vi "處理次數.vi"() -> ()   [LabVIEW 2015]
uses:
  <vilib>/vision/NI_Vision_Development_Module.lvlib
panel:
  out "Count":i32
  in  "Gap":i32=10 min=1 max=300
  in  "Direction":T1(ring)
  in  "Rectangle Points":T2[](array[typedef]) {"Y" format="%.2f"; "X" format="%.2f"}
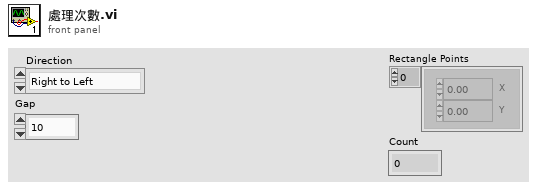
[diagram p1: front panel]
types:
  T1 = enum16{"Right to Left", "Left  to Right", "Up to Down", "Down to Up"}
  T2 = typedef "IMAQ Point" = cluster{"X":sgl, "Y":sgl}
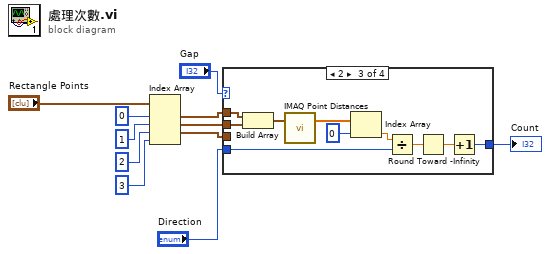
[diagram p0: block diagram]
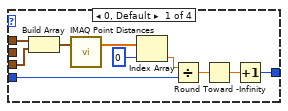
[diagram p2: hidden frame]
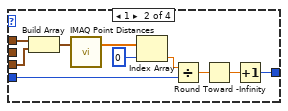
[diagram p3: hidden frame]
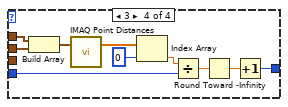
[diagram p4: hidden frame]
diagram:
  n1 = Index Array(array="Rectangle Points", index #1=0 ("index"), index #2=1 ("index"), index #3=2 ("index"), index #4=3 ("index")) -> (element #1=w6:T2, element #2=w4:T2, element #3=w5:T2)  [unwired: 1 out]
  n2 = case shown="2" "Gap" {
    tunnel: "Direction" -> [w19 w29 w39 w49]
    tunnel: [w18 w28 w38 w48] -> w1
    tunnel: w6 -> [w15 w25 w37 w45]
    tunnel: w5 -> [w14 w24 _ _]
    tunnel: w4 -> [_ _ w33 w44]
    frame 0, Default {
      n3 = Build Array(w15, w14) -> (w17:T2[])
      n4 = call "IMAQ Point Distances"("Points"=w17) -> ("Distances"=w16:sgl[])  [unwired: 4 in, 1 out]
      n5 = Index Array(array=w16, index=0) -> (element=w12:sgl)
      n6 = Divide(x=w12, y=w19) -> (x/y=w20:sgl)
      n7 = Round Toward -Infinity(1:w20) -> (0:w21:sgl)
      n8 = Increment(x=w21) -> (x+1=w18:i32)
    }
    frame 1 {
      n9 = Build Array(w25, w24) -> (w27:T2[])
      n10 = call "IMAQ Point Distances"("Points"=w27) -> ("Distances"=w26:sgl[])  [unwired: 4 in, 1 out]
      n11 = Index Array(array=w26, index=0) -> (element=w22:sgl)
      n12 = Divide(x=w22, y=w29) -> (x/y=w30:sgl)
      n13 = Round Toward -Infinity(1:w30) -> (0:w31:sgl)
      n14 = Increment(x=w31) -> (x+1=w28:i32)
    }
    frame 2 {
      n15 = Build Array(w37, w33) -> (w36:T2[])
      n16 = call "IMAQ Point Distances"("Points"=w36) -> ("Distances"=w35:sgl[])  [unwired: 4 in, 1 out]
      n17 = Index Array(array=w35, index=0) -> (element=w34:sgl)
      n18 = Divide(x=w34, y=w39) -> (x/y=w40:sgl)
      n19 = Round Toward -Infinity(1:w40) -> (0:w41:sgl)
      n20 = Increment(x=w41) -> (x+1=w38:i32)
    }
    frame 3 {
      n21 = Build Array(w45, w44) -> (w47:T2[])
      n22 = call "IMAQ Point Distances"("Points"=w47) -> ("Distances"=w46:sgl[])  [unwired: 4 in, 1 out]
      n23 = Index Array(array=w46, index=0) -> (element=w43:sgl)
      n24 = Divide(x=w43, y=w49) -> (x/y=w50:sgl)
      n25 = Round Toward -Infinity(1:w50) -> (0:w51:sgl)
      n26 = Increment(x=w51) -> (x+1=w48:i32)
    }
  }
  "Count" <- w1
